vi "test-Mecanum-Kinematics-Test1.vi"() -> (3 "All tests passed":bool)   [LabVIEW 2019]
uses:
  <vilib>/Rock Robotics/WPI/ThirdParty/JAS_Junk/TrajLib/Trajectory_Library.lvlib
panel:
  out "Test 13":bool
  out "Test 12":bool
  out "Test 11":bool
  out "Test 10":bool
  out "Test 9":bool
  out "Test 8":bool
  out "Test 7":bool
  out "Test 6":bool
  out "Test 5":bool
  out "Test 4":bool
  out "Test 3":bool
  out "Test 2":bool
  out "Test 1":bool
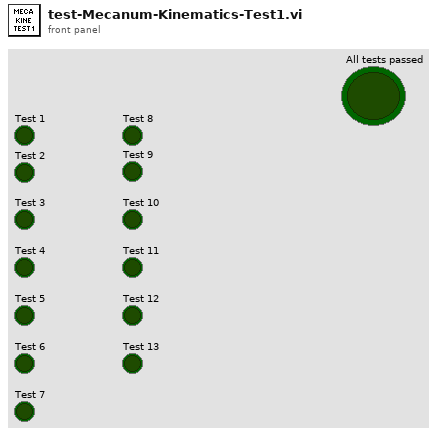
[diagram p1: front panel]
types:
  T1 = typedef "Trajectory_Library.lvlib/TRANSLATION2D.ctl" = cluster{"X":dbl, "Y":dbl}
  T2 = typedef "Trajectory_Library.lvlib/MECA_WHEEL_SPEEDS.ctl" = cluster{"FrontLeftSpeed":dbl, "FrontRightSpeed":dbl, "RearLeftSpeed":dbl, "RearRightSpeed":dbl}
  T3 = typedef "Trajectory_Library.lvlib/CHASSIS_SPEEDS.ctl" = cluster{"vX":dbl, "vY":dbl, "vOmega":dbl}
  T4 = typedef "Trajectory_Library.lvlib/MECA_DRIVE_KINEMATICS.ctl" = cluster{"FrontLeft":T1, "FrontRight":T1, "RearLeft":T1, "RearRight":T1, "InverseKinematics":T5, "ForwardKinematics":T5, "PrevCoR":T1}
  T5 = typedef "NI_Matrix.lvlib/RealMatrix.ctl" = dbl[][]
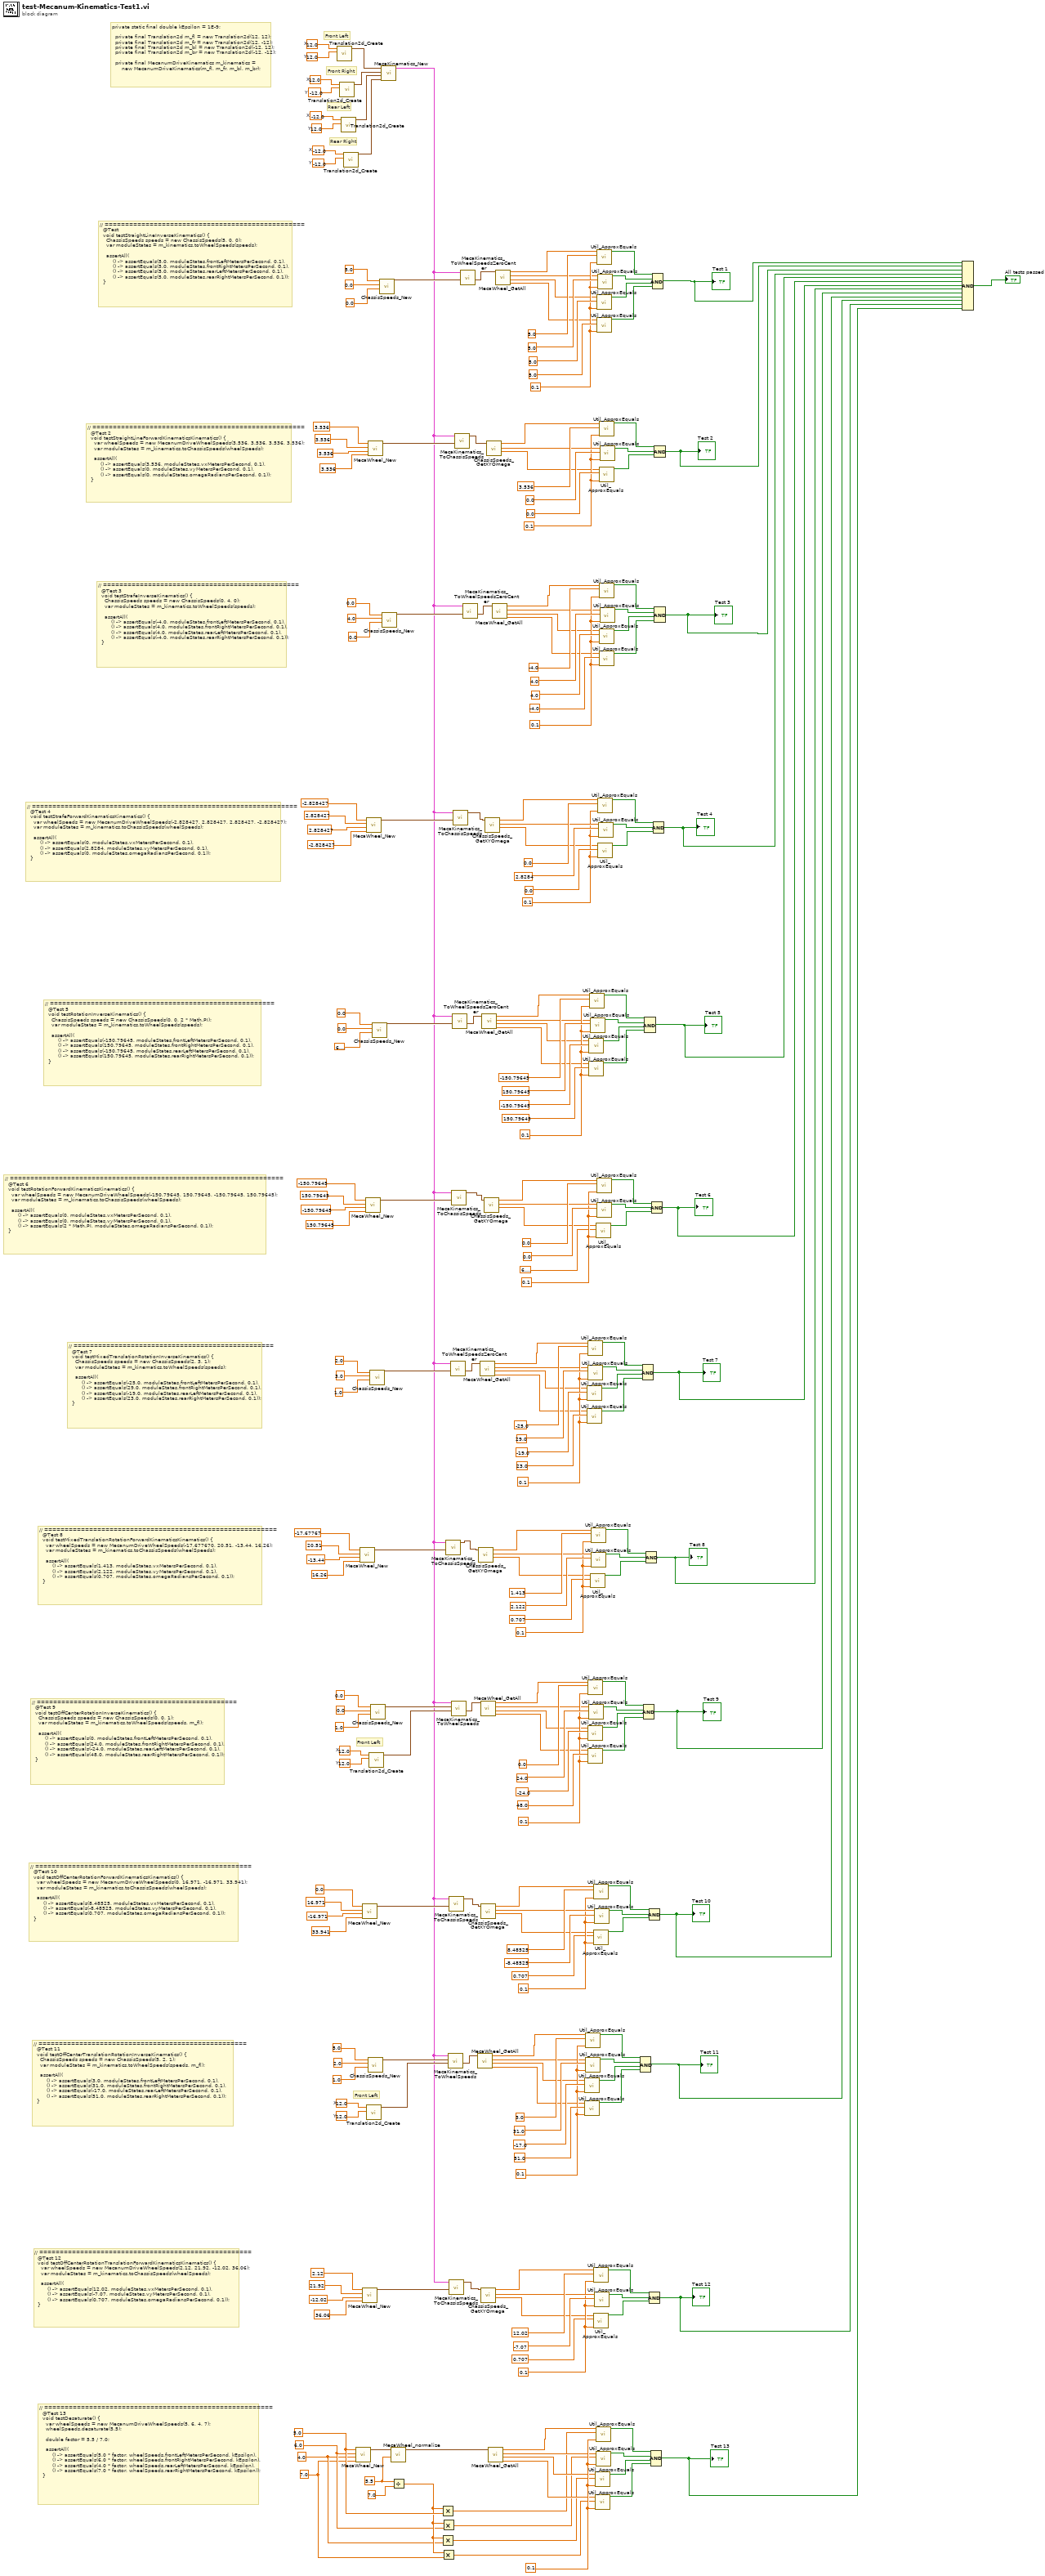
[diagram p0: block diagram]
diagram:
  w17 = 0.1 ("Tolerance")
  w28 = 5.5 ("MaxAttainableSpeed")
  w26 = 5.0 ("FrontLeftSpeed")
  w24 = 6.0 ("FrontRightSpeed")
  w23 = 4.0 ("RearLeftSpeed")
  w22 = 7.0 ("RearRightSpeed")
  w36 = 0.1 ("Tolerance")
  w51 = 12.0  # X
  w49 = 12.0  # Y
  w58 = 0.1 ("Tolerance")
  w72 = 0.1 ("Tolerance")
  w88 = 12.0  # X
  w86 = 12.0  # Y
  w95 = 0.1 ("Tolerance")
  w115 = 0.1 ("Tolerance")
  w134 = 0.1 ("Tolerance")
  w148 = 0.1 ("Tolerance")
  w167 = 0.1 ("Tolerance")
  w180 = 0.1 ("Tolerance")
  w205 = 0.1 ("Tolerance")
  w206 = 0.1 ("Tolerance")
  w207 = 0.1 ("Tolerance")
  w251 = -12.0  # X
  w250 = -12.0  # Y
  w249 = -12.0  # X
  w248 = 12.0  # Y
  w247 = 12.0  # X
  w246 = -12.0  # Y
  w245 = 12.0  # X
  w244 = 12.0  # Y
  # "// ========================================================\n  @Test 13\n  void testDesaturate() {\n    var wheelSpeeds = new MecanumDriveWheelSpeeds(5, 6, 4, 7);\n    wheelSpeeds.desaturate(5.5);\n\n    double factor = 5.5 / 7.0;\n\n    assertAll(\n        () -> assertEquals(5.0 * factor, wheelSpeeds.frontLeftMetersPerSecond, kEpsilon),\n        () -> assertEquals(6.0 * factor, wheelSpeeds.frontRightMetersPerSecond, kEpsilon),\n        () -> assertEquals(4.0 * factor, wheelSpeeds.rearLeftMetersPerSecond, kEpsilon),\n        () -> assertEquals(7.0 * factor, wheelSpeeds.rearRightMetersPerSecond, kEpsilon));\n  }"
  # "// ====================================================\n  @Test 12\n  void testOffCenterRotationTranslationForwardKinematicsKinematics() {\n    var wheelSpeeds = new MecanumDriveWheelSpeeds(2.12, 21.92, -12.02, 36.06);\n    var moduleStates = m_kinematics.toChassisSpeeds(wheelSpeeds);\n\n    assertAll(\n        () -> assertEquals(12.02, moduleStates.vxMetersPerSecond, 0.1),\n        () -> assertEquals(-7.07, moduleStates.vyMetersPerSecond, 0.1),\n        () -> assertEquals(0.707, moduleStates.omegaRadiansPerSecond, 0.1));\n  }"
  # "// ===================================================\n  @Test 11\n  void testOffCenterTranslationRotationInverseKinematics() {\n    ChassisSpeeds speeds = new ChassisSpeeds(5, 2, 1);\n    var moduleStates = m_kinematics.toWheelSpeeds(speeds, m_fl);\n\n    assertAll(\n        () -> assertEquals(3.0, moduleStates.frontLeftMetersPerSecond, 0.1),\n        () -> assertEquals(31.0, moduleStates.frontRightMetersPerSecond, 0.1),\n        () -> assertEquals(-17.0, moduleStates.rearLeftMetersPerSecond, 0.1),\n        () -> assertEquals(51.0, moduleStates.rearRightMetersPerSecond, 0.1));\n  }"
  # "Front Left"
  # "// =====================================================\n  @Test 10\n  void testOffCenterRotationForwardKinematicsKinematics() {\n    var wheelSpeeds = new MecanumDriveWheelSpeeds(0, 16.971, -16.971, 33.941);\n    var moduleStates = m_kinematics.toChassisSpeeds(wheelSpeeds);\n\n    assertAll(\n        () -> assertEquals(8.48525, moduleStates.vxMetersPerSecond, 0.1),\n        () -> assertEquals(-8.48525, moduleStates.vyMetersPerSecond, 0.1),\n        () -> assertEquals(0.707, moduleStates.omegaRadiansPerSecond, 0.1));\n  }"
  # "Front Left"
  # "// =================================================\n  @Test 9\n  void testOffCenterRotationInverseKinematics() {\n    ChassisSpeeds speeds = new ChassisSpeeds(0, 0, 1);\n    var moduleStates = m_kinematics.toWheelSpeeds(speeds, m_fl);\n\n    assertAll(\n        () -> assertEquals(0, moduleStates.frontLeftMetersPerSecond, 0.1),\n        () -> assertEquals(24.0, moduleStates.frontRightMetersPerSecond, 0.1),\n        () -> assertEquals(-24.0, moduleStates.rearLeftMetersPerSecond, 0.1),\n        () -> assertEquals(48.0, moduleStates.rearRightMetersPerSecond, 0.1));\n  }"
  # "// =========================================================\n  @Test 8\n  void testMixedTranslationRotationForwardKinematicsKinematics() {\n    var wheelSpeeds = new MecanumDriveWheelSpeeds(-17.677670, 20.51, -13.44, 16.26);\n    var moduleStates = m_kinematics.toChassisSpeeds(wheelSpeeds);\n\n    assertAll(\n        () -> assertEquals(1.413, moduleStates.vxMetersPerSecond, 0.1),\n        () -> assertEquals(2.122, moduleStates.vyMetersPerSecond, 0.1),\n        () -> assertEquals(0.707, moduleStates.omegaRadiansPerSecond, 0.1));\n  }"
  # "// =================================================\n  @Test 7\n  void testMixedTranslationRotationInverseKinematics() {\n    ChassisSpeeds speeds = new ChassisSpeeds(2, 3, 1);\n    var moduleStates = m_kinematics.toWheelSpeeds(speeds);\n\n    assertAll(\n        () -> assertEquals(-25.0, moduleStates.frontLeftMetersPerSecond, 0.1),\n        () -> assertEquals(29.0, moduleStates.frontRightMetersPerSecond, 0.1),\n        () -> assertEquals(-19.0, moduleStates.rearLeftMetersPerSecond, 0.1),\n        () -> assertEquals(23.0, moduleStates.rearRightMetersPerSecond, 0.1));\n  }"
  # "// ===================================================================\n  @Test 6\n  void testRotationForwardKinematicsKinematics() {\n    var wheelSpeeds = new MecanumDriveWheelSpeeds(-150.79645, 150.79645, -150.79645, 150.79645);\n    var moduleStates = m_kinematics.toChassisSpeeds(wheelSpeeds);\n\n    assertAll(\n        () -> assertEquals(0, moduleStates.vxMetersPerSecond, 0.1),\n        () -> assertEquals(0, moduleStates.vyMetersPerSecond, 0.1),\n        () -> assertEquals(2 * Math.PI, moduleStates.omegaRadiansPerSecond, 0.1));\n  }"
  # "// =======================================================\n  @Test 5\n  void testRotationInverseKinematics() {\n    ChassisSpeeds speeds = new ChassisSpeeds(0, 0, 2 * Math.PI);\n    var moduleStates = m_kinematics.toWheelSpeeds(speeds);\n\n    assertAll(\n        () -> assertEquals(-150.79645, moduleStates.frontLeftMetersPerSecond, 0.1),\n        () -> assertEquals(150.79645, moduleStates.frontRightMetersPerSecond, 0.1),\n        () -> assertEquals(-150.79645, moduleStates.rearLeftMetersPerSecond, 0.1),\n        () -> assertEquals(150.79645, moduleStates.rearRightMetersPerSecond, 0.1));\n  }"
  # "// =================================================================\n  @Test 4\n  void testStrafeForwardKinematicsKinematics() {\n    var wheelSpeeds = new MecanumDriveWheelSpeeds(-2.828427, 2.828427, 2.828427, -2.828427);\n    var moduleStates = m_kinematics.toChassisSpeeds(wheelSpeeds);\n\n    assertAll(\n        () -> assertEquals(0, moduleStates.vxMetersPerSecond, 0.1),\n        () -> assertEquals(2.8284, moduleStates.vyMetersPerSecond, 0.1),\n        () -> assertEquals(0, moduleStates.omegaRadiansPerSecond, 0.1));\n  }"
  # "// ================================================\n  @Test 3\n  void testStrafeInverseKinematics() {\n    ChassisSpeeds speeds = new ChassisSpeeds(0, 4, 0);\n    var moduleStates = m_kinematics.toWheelSpeeds(speeds);\n\n    assertAll(\n        () -> assertEquals(-4.0, moduleStates.frontLeftMetersPerSecond, 0.1),\n        () -> assertEquals(4.0, moduleStates.frontRightMetersPerSecond, 0.1),\n        () -> assertEquals(4.0, moduleStates.rearLeftMetersPerSecond, 0.1),\n        () -> assertEquals(-4.0, moduleStates.rearRightMetersPerSecond, 0.1));\n  }"
  # "// ====================================================\n  @Test 2\n  void testStraightLineForwardKinematicsKinematics() {\n    var wheelSpeeds = new MecanumDriveWheelSpeeds(3.536, 3.536, 3.536, 3.536);\n    var moduleStates = m_kinematics.toChassisSpeeds(wheelSpeeds);\n\n    assertAll(\n        () -> assertEquals(3.536, moduleStates.vxMetersPerSecond, 0.1),\n        () -> assertEquals(0, moduleStates.vyMetersPerSecond, 0.1),\n        () -> assertEquals(0, moduleStates.omegaRadiansPerSecond, 0.1));\n  }"
  # "Rear Right"
  # "Rear Left"
  # "Front Right"
  # "Front Left"
  # "private static final double kEpsilon = 1E-9;\n\n  private final Translation2d m_fl = new Translation2d(12, 12);\n  private final Translation2d m_fr = new Translation2d(12, -12);\n  private final Translation2d m_bl = new Translation2d(-12, 12);\n  private final Translation2d m_br = new Translation2d(-12, -12);\n\n  private final MecanumDriveKinematics m_kinematics =\n      new MecanumDriveKinematics(m_fl, m_fr, m_bl, m_br);"
  # "// =================================================\n  @Test\n  void testStraightLineInverseKinematics() {\n    ChassisSpeeds speeds = new ChassisSpeeds(5, 0, 0);\n    var moduleStates = m_kinematics.toWheelSpeeds(speeds);\n\n    assertAll(\n        () -> assertEquals(5.0, moduleStates.frontLeftMetersPerSecond, 0.1),\n        () -> assertEquals(5.0, moduleStates.frontRightMetersPerSecond, 0.1),\n        () -> assertEquals(5.0, moduleStates.rearLeftMetersPerSecond, 0.1),\n        () -> assertEquals(5.0, moduleStates.rearRightMetersPerSecond, 0.1));\n  }"
  n1 = call <vilib>:"Translation2d_Create.vi"("Y"=w244, "X"=w245) -> ("TRANSLATION"=w252:T1)  [unwired: 9 in]
  n2 = call <vilib>:"Translation2d_Create.vi"("Y"=w246, "X"=w247) -> ("TRANSLATION"=w253:T1)  [unwired: 9 in]
  n3 = call <vilib>:"Translation2d_Create.vi"("Y"=w248, "X"=w249) -> ("TRANSLATION"=w254:T1)  [unwired: 9 in]
  n4 = call <vilib>:"Translation2d_Create.vi"("Y"=w250, "X"=w251) -> ("TRANSLATION"=w255:T1)  [unwired: 9 in]
  n5 = call <vilib>:"MecaWheel_New.vi"("RearRightSpeed"=w22, "RearLeftSpeed"=w23, "FrontRightSpeed"=w24, "FrontLeftSpeed"=w26) -> ("MECA_WHEEL_SPEEDS"=w29:T2)  [unwired: 7 in]
  n6 = call <vilib>:"MecaWheel_New.vi"("RearRightSpeed"=16.26, "RearLeftSpeed"=-13.44, "FrontRightSpeed"=20.51, "FrontLeftSpeed"=-17.67767) -> ("MECA_WHEEL_SPEEDS"=w118:T2)  [unwired: 7 in]
  n7 = call <vilib>:"MecaWheel_New.vi"("RearRightSpeed"=33.941, "RearLeftSpeed"=-16.971, "FrontRightSpeed"=16.971, "FrontLeftSpeed"=0.0) -> ("MECA_WHEEL_SPEEDS"=w75:T2)  [unwired: 7 in]
  n8 = call <vilib>:"MecaWheel_New.vi"("RearRightSpeed"=36.06, "RearLeftSpeed"=-12.02, "FrontRightSpeed"=21.92, "FrontLeftSpeed"=2.12) -> ("MECA_WHEEL_SPEEDS"=w39:T2)  [unwired: 7 in]
  n9 = call <vilib>:"MecaWheel_New.vi"("RearRightSpeed"=150.79645, "RearLeftSpeed"=-150.79645, "FrontRightSpeed"=150.79645, "FrontLeftSpeed"=-150.79645) -> ("MECA_WHEEL_SPEEDS"=w151:T2)  [unwired: 7 in]
  n10 = call <vilib>:"Translation2d_Create.vi"("Y"=w49, "X"=w51) -> ("TRANSLATION"=w50:T1)  [unwired: 9 in]
  n11 = call <vilib>:"MecaWheel_New.vi"("RearRightSpeed"=-2.828427, "RearLeftSpeed"=2.828427, "FrontRightSpeed"=2.828427, "FrontLeftSpeed"=-2.828427) -> ("MECA_WHEEL_SPEEDS"=w183:T2)  [unwired: 7 in]
  n12 = call <vilib>:"ChassisSpeeds_New.vi"("vAngular"=1.0 ("vX"), "vY"=2.0, "vX"=5.0) -> ("CHASSIS"=w33:T3)  [unwired: 8 in]
  n13 = call <vilib>:"MecaWheel_New.vi"("RearRightSpeed"=3.536, "RearLeftSpeed"=3.536, "FrontRightSpeed"=3.536, "FrontLeftSpeed"=3.536) -> ("MECA_WHEEL_SPEEDS"=w223:T2)  [unwired: 7 in]
  n14 = call <vilib>:"Translation2d_Create.vi"("Y"=w86, "X"=w88) -> ("TRANSLATION"=w87:T1)  [unwired: 9 in]
  n15 = call <vilib>:"ChassisSpeeds_New.vi"("vAngular"=1.0 ("vX"), "vY"=3.0, "vX"=2.0) -> ("CHASSIS"=w143:T3)  [unwired: 8 in]
  n16 = call <vilib>:"ChassisSpeeds_New.vi"("vAngular"=1.0 ("vX"), "vY"=0.0, "vX"=0.0) -> ("CHASSIS"=w104:T3)  [unwired: 8 in]
  n17 = call <vilib>:"ChassisSpeeds_New.vi"("vAngular"=6.283185307179586, "vY"=0.0, "vX"=0.0) -> ("CHASSIS"=w176:T3)  [unwired: 8 in]
  n18 = call <vilib>:"ChassisSpeeds_New.vi"("vAngular"=0.0, "vY"=0.0, "vX"=5.0) -> ("CHASSIS"=w243:T3)  [unwired: 8 in]
  n19 = call <vilib>:"MecaKinematics_New.vi"("RearRight"=w255, "RearLeft"=w254, "FrontRight"=w253, "FrontLeft"=w252) -> ("MECA_DRIVE_KINEMATICS"=w32:T4)  [unwired: 7 in]
  n20 = call <vilib>:"ChassisSpeeds_New.vi"("vAngular"=0.0, "vY"=4.0, "vX"=0.0) -> ("CHASSIS"=w216:T3)  [unwired: 8 in]
  n21 = call <vilib>:"MecaWheel_normalize.vi"("MaxAttainableSpeed"=w28, "in MECA_WHEEL_SPEEDS"=w29) -> ("out MECA_WHEEL_SPEEDS"=w12:T2)  [unwired: 9 in]
  n22 = Divide(x=w28, y=7.0) -> (x/y=w25:dbl)
  n23 = Multiply(x=w25, y=w26) -> (x*y=w11:dbl)
  n24 = Multiply(x=w25, y=w23) -> (x*y=w9:dbl)
  n25 = Multiply(x=w25, y=w24) -> (x*y=w10:dbl)
  n26 = Multiply(x=w25, y=w22) -> (x*y=w8:dbl)
  n27 = call <vilib>:"MecaKinematics_ToChassisSpeeds.vi"("MECA_WHEEL_SPEEDS"=w118, "in MECA_DRIVE_KINEMATICS"=w32) -> ("ChassisSpeeds"=w4:T3)  [unwired: 9 in]
  n28 = call <vilib>:"MecaKinematics_ToWheelSpeeds.vi"("CenterOfRotation"=w50, "ChassisSpeeds"=w33, "in MECA_DRIVE_KINEMATICS"=w32) -> ("MECA_WHEEL_SPEEDS"=w57:T2)  [unwired: 7 in, 1 out]
  n29 = call <vilib>:"MecaKinematics_ToChassisSpeeds.vi"("MECA_WHEEL_SPEEDS"=w75, "in MECA_DRIVE_KINEMATICS"=w32) -> ("ChassisSpeeds"=w3:T3)  [unwired: 9 in]
  n30 = call <vilib>:"MecaKinematics_ToChassisSpeeds.vi"("MECA_WHEEL_SPEEDS"=w39, "in MECA_DRIVE_KINEMATICS"=w32) -> ("ChassisSpeeds"=w2:T3)  [unwired: 9 in]
  n31 = call <vilib>:"MecaKinematics_ToWheelSpeedsZeroCenter.vi"("ChassisSpeeds"=w143, "in MECA_DRIVE_KINEMATICS"=w32) -> ("MECA_WHEEL_SPEEDS"=w133:T2)  [unwired: 8 in, 1 out]
  n32 = call <vilib>:"MecaKinematics_ToWheelSpeeds.vi"("CenterOfRotation"=w87, "ChassisSpeeds"=w104, "in MECA_DRIVE_KINEMATICS"=w32) -> ("MECA_WHEEL_SPEEDS"=w94:T2)  [unwired: 7 in, 1 out]
  n33 = call <vilib>:"MecaKinematics_ToChassisSpeeds.vi"("MECA_WHEEL_SPEEDS"=w151, "in MECA_DRIVE_KINEMATICS"=w32) -> ("ChassisSpeeds"=w5:T3)  [unwired: 9 in]
  n34 = call <vilib>:"MecaKinematics_ToWheelSpeedsZeroCenter.vi"("ChassisSpeeds"=w176, "in MECA_DRIVE_KINEMATICS"=w32) -> ("MECA_WHEEL_SPEEDS"=w166:T2)  [unwired: 8 in, 1 out]
  n35 = call <vilib>:"MecaKinematics_ToChassisSpeeds.vi"("MECA_WHEEL_SPEEDS"=w183, "in MECA_DRIVE_KINEMATICS"=w32) -> ("ChassisSpeeds"=w1:T3)  [unwired: 9 in]
  n36 = call <vilib>:"MecaKinematics_ToChassisSpeeds.vi"("MECA_WHEEL_SPEEDS"=w223, "in MECA_DRIVE_KINEMATICS"=w32) -> ("ChassisSpeeds"=w6:T3)  [unwired: 9 in]
  n37 = call <vilib>:"MecaKinematics_ToWheelSpeedsZeroCenter.vi"("ChassisSpeeds"=w243, "in MECA_DRIVE_KINEMATICS"=w32) -> ("MECA_WHEEL_SPEEDS"=w204:T2)  [unwired: 8 in, 1 out]
  n38 = call <vilib>:"MecaKinematics_ToWheelSpeedsZeroCenter.vi"("ChassisSpeeds"=w216, "in MECA_DRIVE_KINEMATICS"=w32) -> ("MECA_WHEEL_SPEEDS"=w199:T2)  [unwired: 8 in, 1 out]
  n39 = call <vilib>:"MecaWheel_GetAll.vi"("MECA_WHEEL_SPEEDS"=w57) -> ("RearRightSpeed"=w53:dbl, "RearLeftSpeed"=w54:dbl, "FrontRightSpeed"=w55:dbl, "FrontLeftSpeed"=w56:dbl)  [unwired: 7 in]
  n40 = call <vilib>:"ChassisSpeeds_GetXYOmega.vi"("CHASSIS"=w4) -> ("vAngular"=w114:dbl, "vY"=w116:dbl, "vX"=w117:dbl)  [unwired: 8 in]
  n41 = call <vilib>:"MecaWheel_GetAll.vi"("MECA_WHEEL_SPEEDS"=w133) -> ("RearRightSpeed"=w129:dbl, "RearLeftSpeed"=w130:dbl, "FrontRightSpeed"=w131:dbl, "FrontLeftSpeed"=w132:dbl)  [unwired: 7 in]
  n42 = call <vilib>:"MecaWheel_GetAll.vi"("MECA_WHEEL_SPEEDS"=w94) -> ("RearRightSpeed"=w90:dbl, "RearLeftSpeed"=w91:dbl, "FrontRightSpeed"=w92:dbl, "FrontLeftSpeed"=w93:dbl)  [unwired: 7 in]
  n43 = call <vilib>:"ChassisSpeeds_GetXYOmega.vi"("CHASSIS"=w3) -> ("vAngular"=w71:dbl, "vY"=w73:dbl, "vX"=w74:dbl)  [unwired: 8 in]
  n44 = call <vilib>:"ChassisSpeeds_GetXYOmega.vi"("CHASSIS"=w2) -> ("vAngular"=w35:dbl, "vY"=w37:dbl, "vX"=w38:dbl)  [unwired: 8 in]
  n45 = call <vilib>:"MecaWheel_GetAll.vi"("MECA_WHEEL_SPEEDS"=w166) -> ("RearRightSpeed"=w162:dbl, "RearLeftSpeed"=w163:dbl, "FrontRightSpeed"=w164:dbl, "FrontLeftSpeed"=w165:dbl)  [unwired: 7 in]
  n46 = call <vilib>:"ChassisSpeeds_GetXYOmega.vi"("CHASSIS"=w5) -> ("vAngular"=w147:dbl, "vY"=w149:dbl, "vX"=w150:dbl)  [unwired: 8 in]
  n47 = call <vilib>:"ChassisSpeeds_GetXYOmega.vi"("CHASSIS"=w1) -> ("vAngular"=w179:dbl, "vY"=w181:dbl, "vX"=w182:dbl)  [unwired: 8 in]
  n48 = call <vilib>:"ChassisSpeeds_GetXYOmega.vi"("CHASSIS"=w6) -> ("vAngular"=w194:dbl, "vY"=w221:dbl, "vX"=w222:dbl)  [unwired: 8 in]
  n49 = call <vilib>:"MecaWheel_GetAll.vi"("MECA_WHEEL_SPEEDS"=w12) -> ("RearRightSpeed"=w13:dbl, "RearLeftSpeed"=w14:dbl, "FrontRightSpeed"=w15:dbl, "FrontLeftSpeed"=w16:dbl)  [unwired: 7 in]
  n50 = call <vilib>:"MecaWheel_GetAll.vi"("MECA_WHEEL_SPEEDS"=w199) -> ("RearRightSpeed"=w195:dbl, "RearLeftSpeed"=w196:dbl, "FrontRightSpeed"=w197:dbl, "FrontLeftSpeed"=w198:dbl)  [unwired: 7 in]
  n51 = call <vilib>:"MecaWheel_GetAll.vi"("MECA_WHEEL_SPEEDS"=w204) -> ("RearRightSpeed"=w200:dbl, "RearLeftSpeed"=w201:dbl, "FrontRightSpeed"=w202:dbl, "FrontLeftSpeed"=w203:dbl)  [unwired: 7 in]
  n52 = call <vilib>:"Util_ApproxEquals.vi"("Tolerance"=w58, "Value 2"=-17.0, "Value 1"=w54) -> ("ApproxEquals"=w60:bool)  [unwired: 8 in]
  n53 = call <vilib>:"Util_ApproxEquals.vi"("Tolerance"=w58, "Value 2"=51.0, "Value 1"=w53) -> ("ApproxEquals"=w59:bool)  [unwired: 8 in]
  n54 = call <vilib>:"Util_ApproxEquals.vi"("Tolerance"=w58, "Value 2"=3.0, "Value 1"=w56) -> ("ApproxEquals"=w62:bool)  [unwired: 8 in]
  n55 = call <vilib>:"Util_ApproxEquals.vi"("Tolerance"=w58, "Value 2"=31.0, "Value 1"=w55) -> ("ApproxEquals"=w61:bool)  [unwired: 8 in]
  n56 = call <vilib>:"Util_ApproxEquals.vi"("Tolerance"=w134, "Value 2"=-19.0, "Value 1"=w130) -> ("ApproxEquals"=w136:bool)  [unwired: 8 in]
  n57 = call <vilib>:"Util_ApproxEquals.vi"("Tolerance"=w134, "Value 2"=23.0, "Value 1"=w129) -> ("ApproxEquals"=w135:bool)  [unwired: 8 in]
  n58 = call <vilib>:"Util_ApproxEquals.vi"("Tolerance"=w134, "Value 2"=-25.0, "Value 1"=w132) -> ("ApproxEquals"=w138:bool)  [unwired: 8 in]
  n59 = call <vilib>:"Util_ApproxEquals.vi"("Tolerance"=w95, "Value 2"=-24.0, "Value 1"=w91) -> ("ApproxEquals"=w97:bool)  [unwired: 8 in]
  n60 = call <vilib>:"Util_ApproxEquals.vi"("Tolerance"=w95, "Value 2"=48.0, "Value 1"=w90) -> ("ApproxEquals"=w96:bool)  [unwired: 8 in]
  n61 = call <vilib>:"Util_ApproxEquals.vi"("Tolerance"=w134, "Value 2"=29.0, "Value 1"=w131) -> ("ApproxEquals"=w137:bool)  [unwired: 8 in]
  n62 = call <vilib>:"Util_ApproxEquals.vi"("Tolerance"=w95, "Value 2"=0.0, "Value 1"=w93) -> ("ApproxEquals"=w99:bool)  [unwired: 8 in]
  n63 = call <vilib>:"Util_ApproxEquals.vi"("Tolerance"=w95, "Value 2"=24.0, "Value 1"=w92) -> ("ApproxEquals"=w98:bool)  [unwired: 8 in]
  n64 = call <vilib>:"Util_ApproxEquals.vi"("Tolerance"=w167, "Value 2"=-150.79645, "Value 1"=w163) -> ("ApproxEquals"=w169:bool)  [unwired: 8 in]
  n65 = call <vilib>:"Util_ApproxEquals.vi"("Tolerance"=w167, "Value 2"=150.79645, "Value 1"=w162) -> ("ApproxEquals"=w168:bool)  [unwired: 8 in]
  n66 = call <vilib>:"Util_ApproxEquals.vi"("Tolerance"=w167, "Value 2"=-150.79645, "Value 1"=w165) -> ("ApproxEquals"=w171:bool)  [unwired: 8 in]
  n67 = call <vilib>:"Util_ApproxEquals.vi"("Tolerance"=w167, "Value 2"=150.79645, "Value 1"=w164) -> ("ApproxEquals"=w170:bool)  [unwired: 8 in]
  n68 = call <vilib>:"Util_ApproxEquals.vi"("Tolerance"=w115, "Value 2"=0.707, "Value 1"=w114) -> ("ApproxEquals"=w123:bool)  [unwired: 8 in]
  n69 = call <vilib>:"Util_ApproxEquals.vi"("Tolerance"=w115, "Value 2"=1.413, "Value 1"=w117) -> ("ApproxEquals"=w125:bool)  [unwired: 8 in]
  n70 = call <vilib>:"Util_ApproxEquals.vi"("Tolerance"=w115, "Value 2"=2.122, "Value 1"=w116) -> ("ApproxEquals"=w124:bool)  [unwired: 8 in]
  n71 = call <vilib>:"Util_ApproxEquals.vi"("Tolerance"=w72, "Value 2"=0.707, "Value 1"=w71) -> ("ApproxEquals"=w80:bool)  [unwired: 8 in]
  n72 = call <vilib>:"Util_ApproxEquals.vi"("Tolerance"=w36, "Value 2"=0.707, "Value 1"=w35) -> ("ApproxEquals"=w44:bool)  [unwired: 8 in]
  n73 = call <vilib>:"Util_ApproxEquals.vi"("Tolerance"=w72, "Value 2"=8.48525, "Value 1"=w74) -> ("ApproxEquals"=w82:bool)  [unwired: 8 in]
  n74 = call <vilib>:"Util_ApproxEquals.vi"("Tolerance"=w36, "Value 2"=12.02, "Value 1"=w38) -> ("ApproxEquals"=w46:bool)  [unwired: 8 in]
  n75 = call <vilib>:"Util_ApproxEquals.vi"("Tolerance"=w72, "Value 2"=-8.48525, "Value 1"=w73) -> ("ApproxEquals"=w81:bool)  [unwired: 8 in]
  n76 = call <vilib>:"Util_ApproxEquals.vi"("Tolerance"=w36, "Value 2"=-7.07, "Value 1"=w37) -> ("ApproxEquals"=w45:bool)  [unwired: 8 in]
  n77 = call <vilib>:"Util_ApproxEquals.vi"("Tolerance"=w17, "Value 2"=w9, "Value 1"=w14) -> ("ApproxEquals"=w19:bool)  [unwired: 8 in]
  n78 = call <vilib>:"Util_ApproxEquals.vi"("Tolerance"=w17, "Value 2"=w8, "Value 1"=w13) -> ("ApproxEquals"=w18:bool)  [unwired: 8 in]
  n79 = call <vilib>:"Util_ApproxEquals.vi"("Tolerance"=w17, "Value 2"=w11, "Value 1"=w16) -> ("ApproxEquals"=w21:bool)  [unwired: 8 in]
  n80 = call <vilib>:"Util_ApproxEquals.vi"("Tolerance"=w148, "Value 2"=6.283185307179586, "Value 1"=w147) -> ("ApproxEquals"=w156:bool)  [unwired: 8 in]
  n81 = call <vilib>:"Util_ApproxEquals.vi"("Tolerance"=w17, "Value 2"=w10, "Value 1"=w15) -> ("ApproxEquals"=w20:bool)  [unwired: 8 in]
  n82 = call <vilib>:"Util_ApproxEquals.vi"("Tolerance"=w207, "Value 2"=5.0, "Value 1"=w201) -> ("ApproxEquals"=w236:bool)  [unwired: 8 in]
  n83 = call <vilib>:"Util_ApproxEquals.vi"("Tolerance"=w207, "Value 2"=5.0, "Value 1"=w200) -> ("ApproxEquals"=w235:bool)  [unwired: 8 in]
  n84 = call <vilib>:"Util_ApproxEquals.vi"("Tolerance"=w148, "Value 2"=0.0, "Value 1"=w150) -> ("ApproxEquals"=w158:bool)  [unwired: 8 in]
  n85 = call <vilib>:"Util_ApproxEquals.vi"("Tolerance"=w207, "Value 2"=5.0, "Value 1"=w203) -> ("ApproxEquals"=w238:bool)  [unwired: 8 in]
  n86 = call <vilib>:"Util_ApproxEquals.vi"("Tolerance"=w148, "Value 2"=0.0, "Value 1"=w149) -> ("ApproxEquals"=w157:bool)  [unwired: 8 in]
  n87 = call <vilib>:"Util_ApproxEquals.vi"("Tolerance"=w207, "Value 2"=5.0, "Value 1"=w202) -> ("ApproxEquals"=w237:bool)  [unwired: 8 in]
  n88 = call <vilib>:"Util_ApproxEquals.vi"("Tolerance"=w180, "Value 2"=0.0, "Value 1"=w179) -> ("ApproxEquals"=w188:bool)  [unwired: 8 in]
  n89 = call <vilib>:"Util_ApproxEquals.vi"("Tolerance"=w180, "Value 2"=0.0, "Value 1"=w182) -> ("ApproxEquals"=w190:bool)  [unwired: 8 in]
  n90 = call <vilib>:"Util_ApproxEquals.vi"("Tolerance"=w180, "Value 2"=2.8284, "Value 1"=w181) -> ("ApproxEquals"=w189:bool)  [unwired: 8 in]
  n91 = call <vilib>:"Util_ApproxEquals.vi"("Tolerance"=w206, "Value 2"=0.0, "Value 1"=w194) -> ("ApproxEquals"=w228:bool)  [unwired: 8 in]
  n92 = call <vilib>:"Util_ApproxEquals.vi"("Tolerance"=w205, "Value 2"=4.0, "Value 1"=w196) -> ("ApproxEquals"=w209:bool)  [unwired: 8 in]
  n93 = call <vilib>:"Util_ApproxEquals.vi"("Tolerance"=w205, "Value 2"=-4.0, "Value 1"=w195) -> ("ApproxEquals"=w208:bool)  [unwired: 8 in]
  n94 = call <vilib>:"Util_ApproxEquals.vi"("Tolerance"=w206, "Value 2"=3.536, "Value 1"=w222) -> ("ApproxEquals"=w230:bool)  [unwired: 8 in]
  n95 = call <vilib>:"Util_ApproxEquals.vi"("Tolerance"=w205, "Value 2"=-4.0, "Value 1"=w198) -> ("ApproxEquals"=w211:bool)  [unwired: 8 in]
  n96 = call <vilib>:"Util_ApproxEquals.vi"("Tolerance"=w206, "Value 2"=0.0, "Value 1"=w221) -> ("ApproxEquals"=w229:bool)  [unwired: 8 in]
  n97 = call <vilib>:"Util_ApproxEquals.vi"("Tolerance"=w205, "Value 2"=4.0, "Value 1"=w197) -> ("ApproxEquals"=w210:bool)  [unwired: 8 in]
  n98 = Compound Arithmetic op=AND(w62, w61, w60, w59) -> (w31:bool)
  "Test 11" <- w31
  n99 = Compound Arithmetic op=AND(w138, w137, w136, w135) -> (w108:bool)
  "Test 7" <- w108
  n100 = Compound Arithmetic op=AND(w99, w98, w97, w96) -> (w85:bool)
  "Test 9" <- w85
  n101 = Compound Arithmetic op=AND(w171, w170, w169, w168) -> (w110:bool)
  "Test 5" <- w110
  n102 = Compound Arithmetic op=AND(w125, w124, w123) -> (w107:bool)
  "Test 8" <- w107
  n103 = Compound Arithmetic op=AND(w82, w81, w80) -> (w69:bool)
  "Test 10" <- w69
  n104 = Compound Arithmetic op=AND(w46, w45, w44) -> (w30:bool)
  "Test 12" <- w30
  n105 = Compound Arithmetic op=AND(w21, w20, w19, w18) -> (w7:bool)
  "Test 13" <- w7
  n106 = Compound Arithmetic op=AND(w158, w157, w156) -> (w109:bool)
  "Test 6" <- w109
  n107 = Compound Arithmetic op=AND(w238, w237, w236, w235) -> (w234:bool)
  "Test 1" <- w234
  n108 = Compound Arithmetic op=AND(w190, w189, w188) -> (w111:bool)
  "Test 4" <- w111
  n109 = Compound Arithmetic op=AND(w230, w229, w228) -> (w220:bool)
  "Test 2" <- w220
  n110 = Compound Arithmetic op=AND(w211, w210, w209, w208) -> (w112:bool)
  "Test 3" <- w112
  n111 = Compound Arithmetic op=AND(w234, w220, w112, w111, w110, w109, w108, w107, w85, w69, w31, w30, w7) -> (→"All tests passed":bool)
